vi "Normal VI.vi"() -> ()   [LabVIEW 2013]
panel:
  in  "Pause":bool
  out "Time Stamp":timestamp format="%<%X\n%x>T"
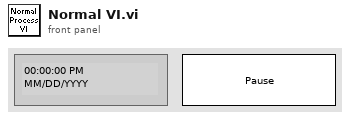
[diagram p1: front panel]
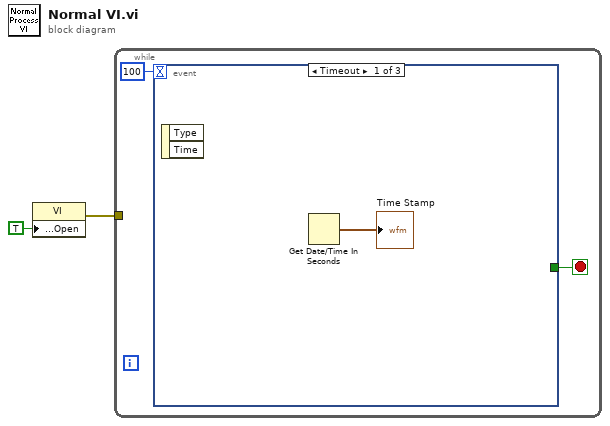
[diagram p0: block diagram]
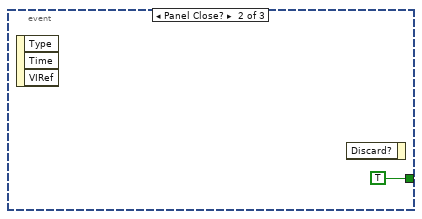
[diagram p2: hidden frame]
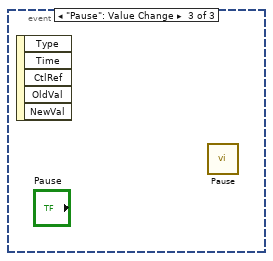
[diagram p3: hidden frame]
diagram:
  n1 = property class="VI"("Front Panel.Open"=TRUE ("Front Panel Window:Open")) -> (error out=w1:errorcluster)  [unwired: 2 in, 1 out]
  n2 = while {
    tunnel: w1 -> [_]
    stop <- w3 stop-if-true
    n3 = event shown="[0] Timeout" {
      selector: _ -> [_ _ _]
      dyn-events: _ -> [_ _ _]
      timeout: 100 -> [_ _ _]
      tunnel: [_ TRUE ("Discard?") _] -> w3
      event Timeout {
        n4 = event-data() -> ()  [unwired: 1 in, 2 out]
        n5 = Get Date/Time In Seconds() -> (seconds since 1Jan1904=→"Time Stamp":timestamp)
      }
      event Panel Close? {
        n6 = event-data() -> ()  [unwired: 1 in, 3 out]
        n7 = event-data() -> ()  [unwired: 2 in, 1 out]
      }
      event "Pause": Value Change {
        n8 = event-data() -> ()  [unwired: 1 in, 5 out]
        n9 = call "Pause.vi"() -> ()  [unwired: 10 in, 2 out]
      }
    }
  }
